vi "GetTimingBySignalName.vi"(10 "Signal Name":string, 11 "Trigger Data":T3) -> (3 "Timing":dbl)   [LabVIEW 2016]
uses:
  Ctrl_Signal.ctl
  Ctrl_Signal_Map.ctl
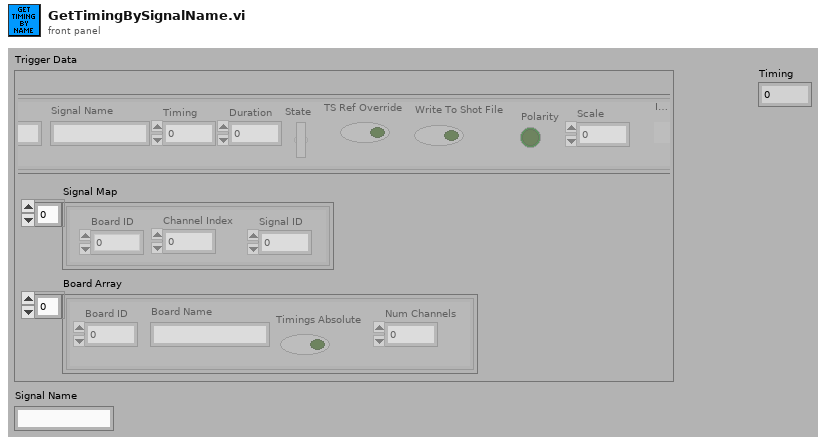
[diagram p1: front panel]
types:
  T1 = typedef "Ctrl_Signal.ctl" = cluster{"Signal Name":string, "Timing":dbl, "Duration":dbl, "State":bool, "TS Ref Override":bool, "Write To Shot File":bool, "Polarity":bool, "Signal ID":dbl, "Scale":dbl, "IsDelay":bool}
  T2 = typedef "Ctrl_Signal_Map.ctl" = cluster{"Channel Index":dbl, "Board ID":dbl, "Signal ID":dbl}
  T3 = cluster{"Signal Array":T1[], "Signal Map":T2[], "Board Array":cluster{"Board ID":dbl, "Board Name":string, "Timings Absolute":bool, "Num Channels":dbl}[]}
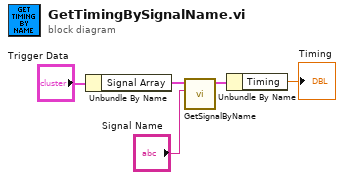
[diagram p0: block diagram]
diagram:
  n1 = Unbundle By Name("Trigger Data") -> ("Signal Array"=w4:T1[])
  n2 = call "GetSignalByName.vi"("Signal Name"="Signal Name", "Signal Array Input"=w4) -> ("Retreived Signal"=w2:T1)  [unwired: 9 in]
  n3 = Unbundle By Name(w2) -> ("Timing"=→"Timing":dbl)
